vi "Compare Two Paths.vi"(4 "Path":path=path "D:/a/b/c/d/e.txt", 5 "Ref Path":path=path "D:/a/b/c/1.xx") -> (0 "different types?":bool, 1 "relative path from 1 to 2":path=path "../d/e.txt", 2 "common path":path=path "D:/a/b/c")   [LabVIEW 2017]
doc: "Compare Two Paths.vi - Compares two paths and if the paths are the same type (both absolute or both relative), the relative path between them is returned."
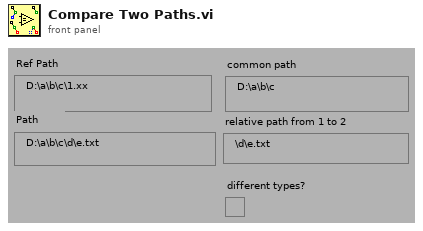
[diagram p1: front panel]
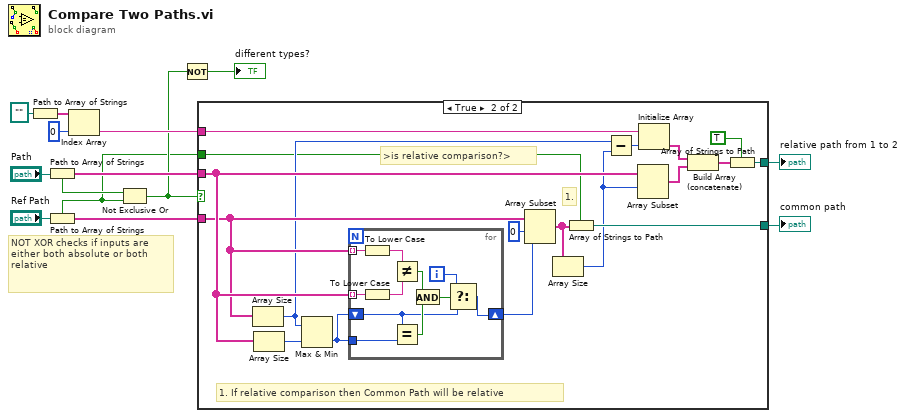
[diagram p0: block diagram]
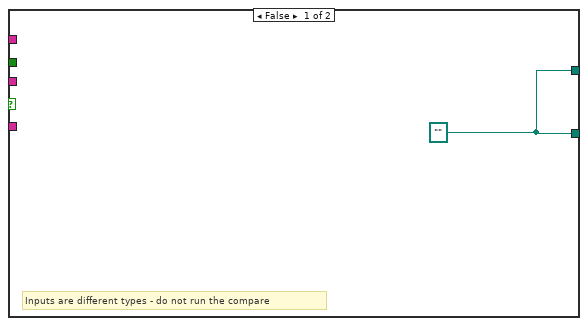
[diagram p2: hidden frame]
diagram:
  # "NOT XOR checks if inputs are either both absolute or both relative"
  n1 = Path to Array of Strings(0:path "..") -> (2:w6:string[])  [unwired: 1 out]
  n2 = Path to Array of Strings(0:"Path") -> (1:w4:bool, 2:w11:string[])
  n3 = Path to Array of Strings(0:"Ref Path") -> (1:w1:bool, 2:w12:string[])
  n4 = Index Array(array=w6, index=0) -> (element=w5:string)
  n5 = Not Exclusive Or(1:w1, 2:w4) -> (0:w3:bool)
  n6 = Not(x=w3) -> (.not. x?=→"different types?":bool)
  n7 = case shown="True" w3 {
    tunnel: w12 -> [_ w21]
    tunnel: w11 -> [_ w26]
    tunnel: [w15 w31] -> w10
    tunnel: [w15 w22] -> w9
    tunnel: w5 -> [_ w28]
    tunnel: w1 -> [_ w16]
    frame False {
      w15 = path "" ("path")
      # "Inputs are different types - do not run the compare"
    }
    frame True {
      # "1."
      # "1. If relative comparison then Common Path will be relative"
      # ">is relative comparison?>"
      n8 = Array Size(array=w21) -> (size(s)=w20:i32)
      n9 = Array Size(array=w26) -> (size(s)=w19:i32)
      n10 = Max & Min(x=w20, y=w19) -> (min(x,y)=w18:i32)  [unwired: 1 out]
      n11 = for {
        tunnel: w21 -> [w44] mode=indexing
        tunnel: w26 -> [w43] mode=indexing
        shift-right: [w36] -> w33
        shift-left: w18 -> [w37]
        tunnel: w18 -> [w42]
        i -> [w38]
        n12 = To Lower Case(string=w44) -> (all lower case string=w35:string)
        n13 = To Lower Case(string=w43) -> (all lower case string=w34:string)
        n14 = Not Equal?(x=w35, y=w34) -> (x != y?=w40:bool)
        n15 = Equal?(x=w37, y=w42) -> (x = y?=w41:bool)
        n16 = And(x=w40, y=w41) -> (x .and. y?=w39:bool)
        n17 = Select(t=w38, s=w39, f=w37) -> (s? t:f=w36:i32)
      }
      n18 = Array Subset(array=w21, index=0, length=w33) -> (w30:string[])
      n19 = Array Size(array=w30) -> (size(s)=w17:i32)
      n20 = Array of Strings to Path(0:w30, 1:w16) -> (2:w31:path)
      n21 = Subtract(x=w20, y=w17) -> (x-y=w29:i32)
      n22 = Array Subset(array=w26, index=w17) -> (w25:string[])  [unwired: 1 in]
      n23 = Initialize Array(w28, w29) -> (w27:string[])
      n24 = Build Array (concatenate)(w27, w25) -> (w24:string[])
      n25 = Array of Strings to Path(0:w24, 1:TRUE ("relative")) -> (2:w22:path)
    }
  }
  "relative path from 1 to 2" <- w9
  "common path" <- w10
